vi "Get Find.vi"(8 "error in (no error)":errorcluster caption="entrée d'erreur (pas d'erreur)", 11 "Find_SN_In_Database en entrée":refnum<class "Find_SN_In_Database.lvclass">) -> (0 "error out":errorcluster caption="sortie d'erreur", 2 "Find":bool, 3 "Find_SN_In_Database en sortie":refnum<class "Find_SN_In_Database.lvclass">)   [LabVIEW 2020, in "Library Test.lvlib" / "Find_SN_In_Database.lvclass"]
uses:
  Find_SN_In_Database.lvclass
  Find_SN_In_Database.lvclass/Find_SN_In_Database.ctl
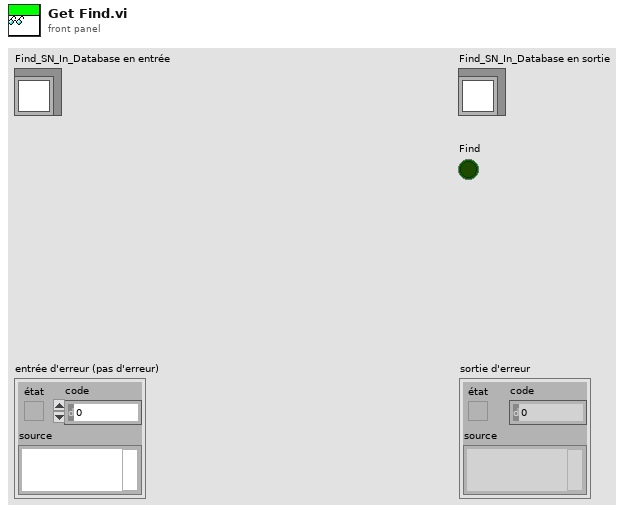
[diagram p1: front panel]
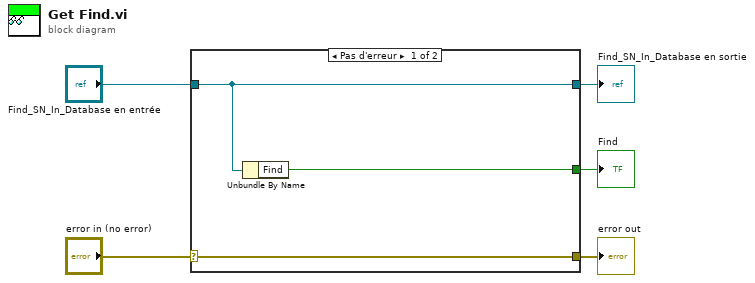
[diagram p0: block diagram]
diagram:
  n1 = case shown="Pas d'erreur" "error in (no error)" {
    selector: "error in (no error)" -> [w8 w9]
    tunnel: [w8 w9] -> w4
    tunnel: [w7 w10] -> w2
    tunnel: "Find_SN_In_Database en entrée" -> [w7 w10]
    tunnel: [w6 _] -> w1
    frame No Error {
      n2 = Unbundle By Name(w7) -> ("Find"=w6:bool)
    }
    frame Error {
    }
  }
  "error out" <- w4
  "Find_SN_In_Database en sortie" <- w2
  "Find" <- w1
